vi "Convolution with I.C..vi"(4 "algorithm":enum32{"direct", "frequency domain"}(ring)=enum."frequency domain", 6 "Initial conditions":dbl[](array[numeric]), 7 "Kernel":dbl[](array[numeric]), 8 "Array in":dbl[](array[numeric])) -> (0 "error":i32, 1 "final conditions":dbl[](array[numeric]), 3 "Array out":dbl[](array[numeric]))   [LabVIEW 2020, in "NI_MAPro.lvlib"]
uses:
  NI_MAPro.lvlib
  NI_AALPro.lvlib
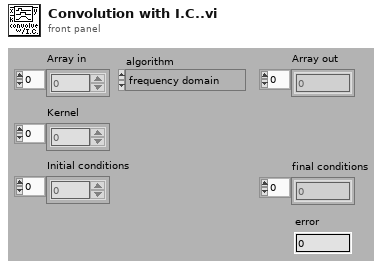
[diagram p1: front panel]
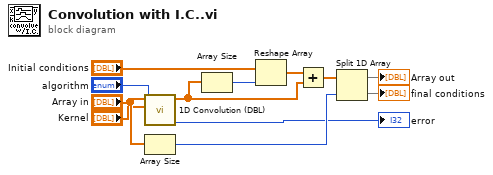
[diagram p0: block diagram]
diagram:
  n1 = call "1D Convolution (DBL).vi"("algorithm"="algorithm", "Y"="Kernel", "X"="Array in") -> ("error"=→"error":i32, "X * Y"=w10:dbl[])  [unwired: 7 in]
  n2 = Array Size(array="Array in") -> (size(s)=w8:i32)
  n3 = Array Size(array=w10) -> (size(s)=w12:i32)
  n4 = Reshape Array("Initial conditions", w12) -> (w11:dbl[])
  n5 = Add(x=w11, y=w10) -> (x+y=w9:dbl[])
  n6 = Split 1D Array(array=w9, index=w8) -> (first subarray=→"Array out":dbl[], second subarray=→"final conditions":dbl[])
